vi "Test Existing Received File is Deleted if Test Passes.vi"(11 "Test Case In":refnum<class "Basic Mechanics Tests.lvclass">) -> (0 "error out":errorcluster, 3 "Test Case Out":refnum<class "Basic Mechanics Tests.lvclass">)   [LabVIEW 2020, in "Basic Mechanics Tests.lvclass"]
uses:
  Basic Mechanics Tests.lvclass
  Source/Approval Tests/Options/Options.lvclass
  Source/Approval Tests/Report Nothing/Report Nothing.lvclass
  Source/Approval Tests/Scrubber/Scrubber.lvclass
  Source/Approval Tests/Namer/Namer.lvclass
  Source/Approval Tests/Naming Data/Naming Data.lvclass
  Source/Approval Tests/Reporter/Reporter.lvclass
  Source/Approval Tests/Text Comparator/Text Comparator.lvclass
  Basic Mechanics Tests.lvclass/Basic Mechanics Tests.ctl
  4be351cf-9afa-44a9-9686-c31d6937e1da.vi
  <vilib>/Astemes/LUnit/Test Case.lvclass
  fbf3a6f1-25d3-4b1a-9ed1-fe282719be7b.vi
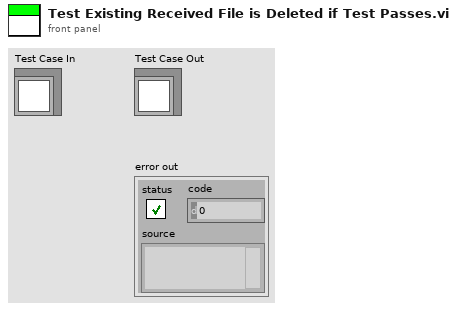
[diagram p1: front panel]
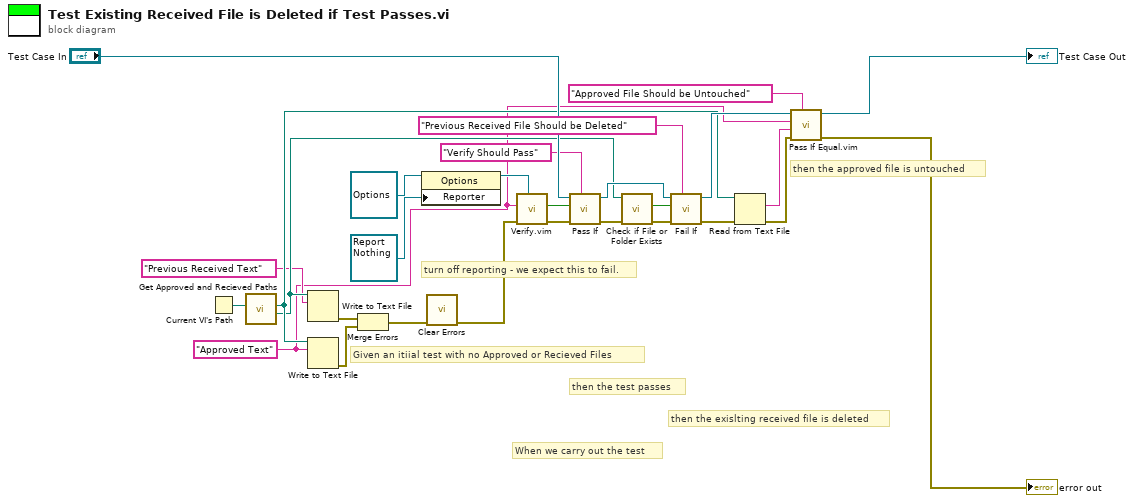
[diagram p0: block diagram]
diagram:
  w5 = "Approved Text"
  # "then the approved file is untouched"
  # "then the exislting received file is deleted"
  # "then the test passes"
  # "When we carry out the test"
  # "Given an itiial test with no Approved or Recieved Files"
  # "turn off reporting - we expect this to fail."
  n1 = Current VI's Path() -> (path=w10:path)
  n2 = call "Get Approved and Recieved Paths.vi"("This VI"=w10) -> ("Recieved"=w7:path, "Approved Path"=w8:path)  [unwired: 9 in]
  n3 = Write to Text File(file (use dialog)=w7, text="Previous Received Text") -> (error out=w20:errorcluster)  [unwired: 2 in, 2 out]
  n4 = Write to Text File(file (use dialog)=w8, text=w5) -> (error out=w21:errorcluster)  [unwired: 2 in, 2 out]
  n5 = Merge Errors(w20, w21) -> (w24:errorcluster)
  n6 = property on="Property Node" class="Options"(reference=refnum<class "Options.lvclass"> refnum ("Options"), "Reporter"=refnum<class "Report Nothing.lvclass"> refnum ("Approval Tests.lvlib:Report Nothing")) -> (reference out=w17:refnum<class "Options.lvclass">)  [unwired: 1 in, 1 out]
  n7 = call <vilib>:"Clear Errors.vi"("error in (no error)"=w24) -> ("error out"=w1:errorcluster)  [unwired: 5 in, 1 out]
  n8 = call "Verify.vim"("Options"=w17, "error in"=w1, "Anything"=w5) -> ("error out"=w25:errorcluster, "Passed?"=w15:bool)  [unwired: 6 in, 1 out]
  n9 = call <vilib>:"Pass If.vi"("Description"="Verify Should Pass", "error in (no error)"=w25, "Pass?"=w15, "LUnit Test Case In"="Test Case In") -> ("error out"=w23:errorcluster, "LUnit Test Case Out"=w14:refnum<class "Basic Mechanics Tests.lvclass">)  [unwired: 6 in]
  n10 = call <vilib>:"Check if File or Folder Exists.vi"("error in (no error)"=w23, "path"=w7) -> ("error out"=w22:errorcluster, "file or folder exists?"=w9:bool)  [unwired: 7 in, 1 out]
  n11 = call <vilib>:"Fail If.vi"("Description"="Previous Received File Should be Deleted", "error in (no error)"=w22, "Fail?"=w9, "LUnit Test Case In"=w14) -> ("error out"=w26:errorcluster, "LUnit Test Case Out"=w13:refnum<class "Basic Mechanics Tests.lvclass">)  [unwired: 6 in]
  n12 = Read from Text File(file (use dialog)=w8, error in=w26) -> (text=w11:string, error out=w27:errorcluster)  [unwired: 2 in, 2 out]
  n13 = call "Pass If Equal.vim"("Description"="Approved File Should be Untouched", "error in (no error)"=w27, "Actual"=w11, "Expected"=w5, "LUnit Test Case In"=w13) -> ("error out"=→"error out":errorcluster, "LUnit Test Case Out"=→"Test Case Out":refnum<class "Basic Mechanics Tests.lvclass">)  [unwired: 5 in]
